vi "Dashboard Main.vi"() -> ()   [LabVIEW 2019]
uses:
  3750-Code-2020-Motion/Motion_Profiler_Class-master/MotionProfile_MP_Class_Status.ctl
  3750-Code-2020-Motion/Motion_Profiler_Class-master/MotionProfile_TalonSetValueEnum.ctl
  <vilib>/Rock Robotics/Network Tables/NT Read Variant.vi
  <vilib>/Rock Robotics/Network Tables/NT Read Number.vi
  <vilib>/Rock Robotics/Network Tables/NT Write Number.vi
  <vilib>/Rock Robotics/Network Tables/NT Write Boolean.vi
  <vilib>/Rock Robotics/Network Tables/NT Write String.vi
  3750-Code-2020-Motion/Motion_Profiler_Class-master/MotionProfiles.lvclass
panel:
  in  "Tab Control":enum32{"MP", "Shooter", "Drivetrain"}(tab)
  in  "Auto Selector":string(combo)
  in  "Start Logging":bool
  out "Right Motor":T1(graph)
  out "Right Throttle":dbl(graph)
  out "Left Throttle":dbl(graph)
  out "Left Motor":T2(graph)
  out "Left Bottom Buf Count":i32
  out "Left Under Run":bool
  out "Right Under Run":bool
  out "Right Bottom Buf Count":i32
  out "Turret Position":cluster{dbl, dbl}(knob) scale=-2000.0..2000.0
  out "Waveform Chart":cluster{"Numeric":dbl, "Numeric":dbl}(graph)
  in  "Set PID":bool
  in  "D":dbl
  in  "I":dbl
  in  "P":dbl
  in  "TCP":refnum<k5>
  out "Robot IP":string
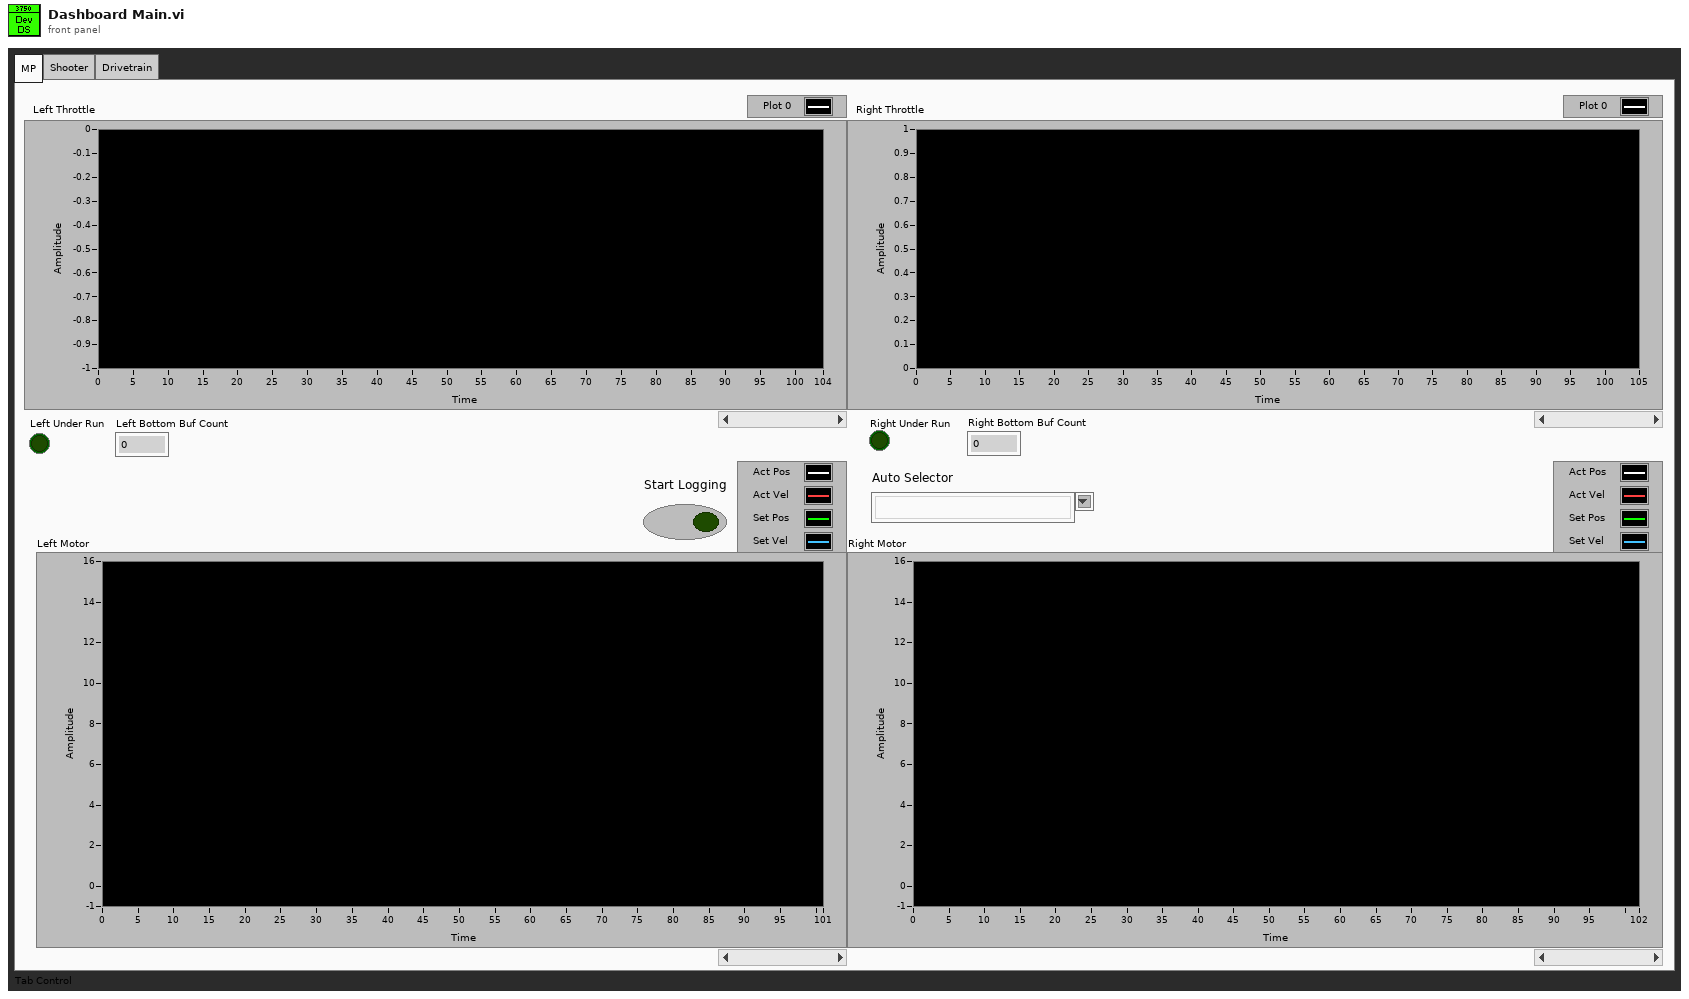
[diagram p1: front panel]
types:
  T1 = cluster{"Set_Vel_(u/100ms)":i32, "Act_Vel_(u/100ms)":i32, "Set_Pos_(u)":i32, "Act_Pos(u)":i32}
  T2 = cluster{"Set_Pos_(u)":i32, "Set_Pos_(u)":i32, "Act_Vel_(u/100ms)":i32, "Set_Vel_(u/100ms)":i32}
  T3 = cluster{"Error Strings":string, "Disable Counts":cluster{u16, u16}, "Rail Faults":cluster{u16, u16, u16}, "Robot IP":string, "DB Mode":u8, "Event Info":cluster{"Name":string, "Type":u8, "Number":u16, "Replay":u8}}
  T4 = cluster{"Storage":cluster{"Disk Free":u64, "RAM Block":u32, "RAM free":u32}, "CPU Utilization":cluster{"CPU % ISR":sgl, "CPU % Time Crit":sgl, "CPU % Timed Str":sgl, "CPU % High":sgl, "CPU % Above":sgl, "CPU % Normal":sgl, "CPU % Low":sgl}, "CAN":cluster{"% Bus Utilization":sgl, "Bus Off Cnt":u32, "TX_FIFO Full Cnt":u32, "Receive Error Cnt":u8, "Transmit Error Cnt":u8}, "HID":cluster{"HID Outputs":u32, "Rumble Low":u16, "Rumble High":u16}[]}
  T5 = cluster{"Status bits":cluster{"Test Mode":bool, "Autonomous":bool, "Enabled":bool, "Code Start":bool, "Brownout":bool, "Reserved 2":bool, "Reserved 3":bool, "E-Stop":bool}, "Code Trace":cluster{"Disabled":bool, "TeleOp":bool, "Auto":bool, "Test":bool}, "Controller Type":enum16{"unknown", "cRIO", "roboRio"}, "Code?":enum16{"unknown", "noCode", "code"}, "Battery V":dbl}
  T6 = cluster{"Control Bits":cluster{"TestMode":bool, "Autonomous":bool, "Enabled":bool, "FMS Present":bool, bool, bool, bool, "E-Stop":bool}, "Team Station ":u8, "Countdown":sgl, "Joystick Values":cluster{"Axes":dbl[], "Buttons":bool[], "POVs":i16[]}[]}
  T7 = enum8{"Tele-Op Disabled", "Tele-Op Enabled", "Auto Disabled", "Auto Enabled", "Test Disabled", "Test Enabled", "Disconnected", "No Code", "E-Stop"}
  T8 = typedef "MotionProfiles.lvclass/MotionProfile_MP_Class_Status.ctl" = cluster{"Motion Profile Status":cluster{"Top Buffer Remaining":i32, "Top Buffer Count":i32, "Bottom Buffer Count":i32, "Has Underrun?":bool, "Is Underrun?":bool, "Active Point Valid?":bool, "Is Last?":bool, "Profile Slot Select 0":i32, "Output Enable":i32, "Time Duration (ms)":i32, "Profile Slot Select 1":i32}, "TalonState":T9, "MP Is Done":bool, "MP Is Executing":bool, "Set_Vel_(u/100ms)":i32, "Set_Pos_(u)":i32, "Act_Vel_(u/100ms)":i32, "Act_Pos(u)":i32, "Throtle":dbl}
  T9 = typedef "MotionProfiles.lvclass/MotionProfile_TalonSetValueEnum.ctl" = enum16{"Disable", "Enable", "Hold"}
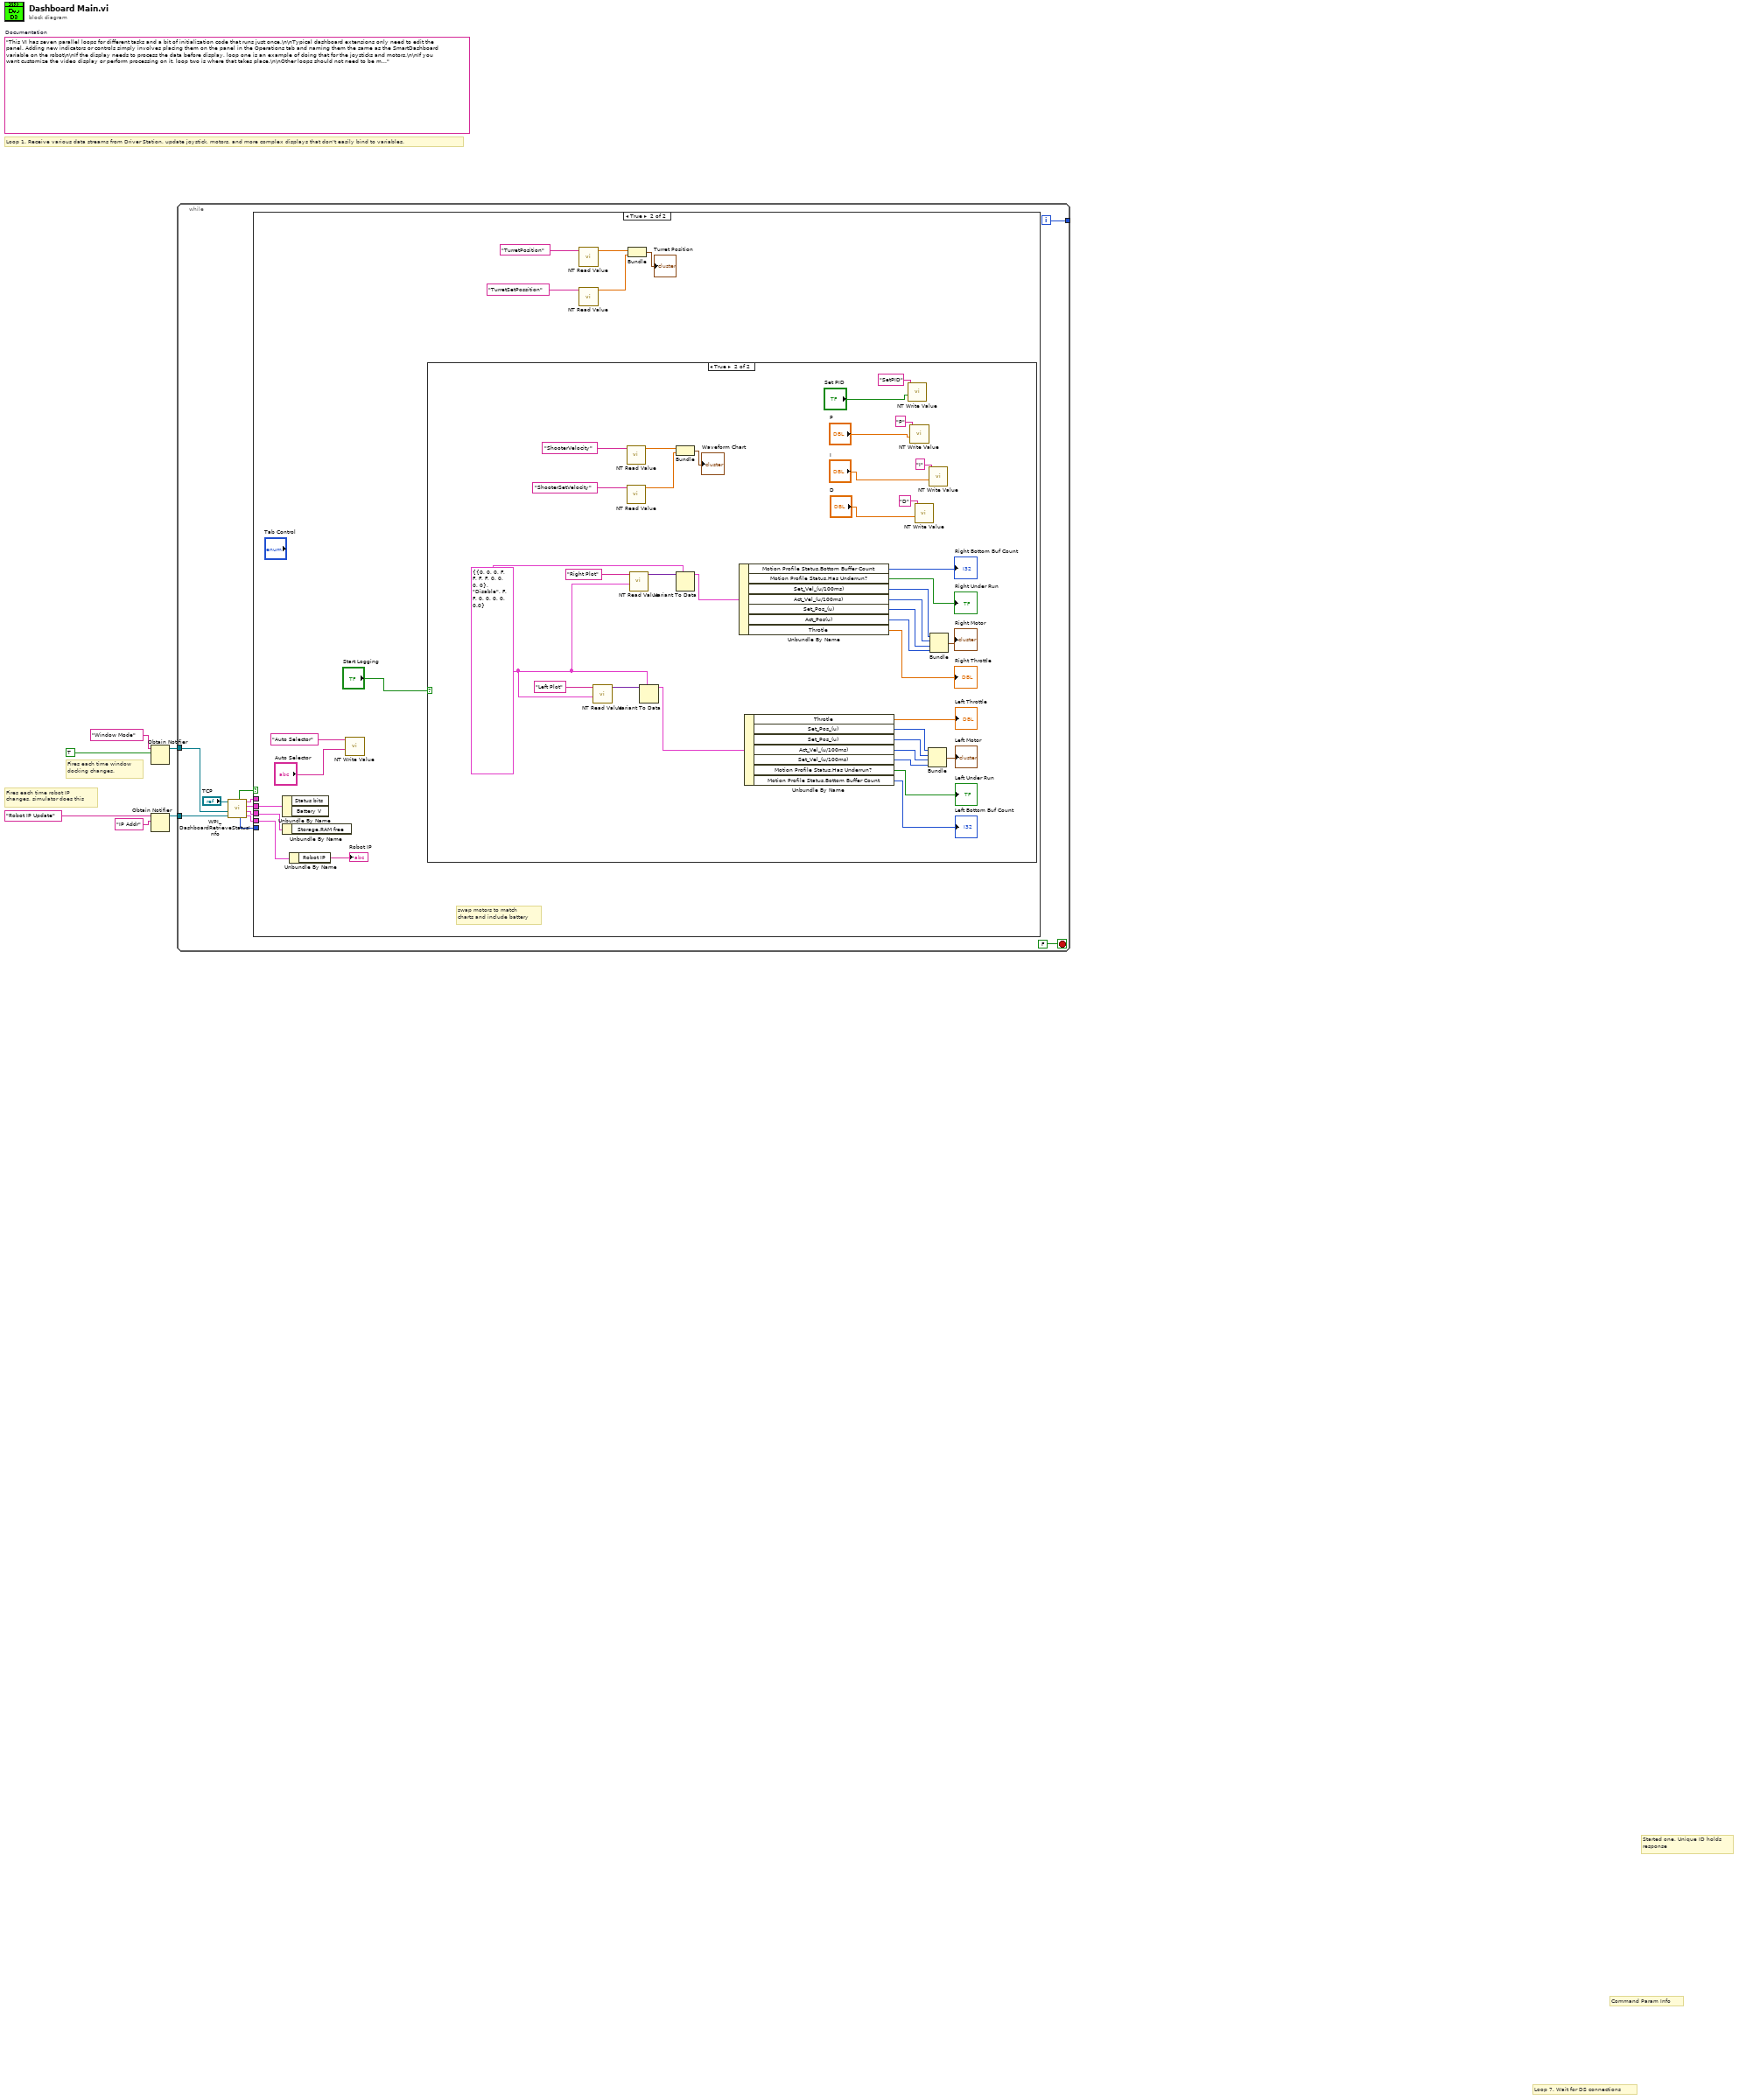
[diagram p0: block diagram]
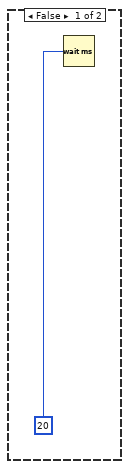
[diagram p2: hidden frame]
diagram:
  (unwired) "This VI has seven parallel loops for different tasks and a bit of initialization code that runs just once.\n\nTypical dashboard extensions only need to edit the panel. Adding new indicators or controls simply involves placing them on the panel in the Operations tab and naming them the same as the SmartDashboard variable on the robot\n\nIf the display needs to process the data before display, loop one is an example of doing that for the joysticks and motors.\n\nIf you want customize the video display or perform processing on it, loop two is where that takes place.\n\nOther loops should not need to be modified. They are pretty standard, and document the task they perform."  # Documentation
  # "Command Param Info"
  # "Started one, Unique ID holds\nresponse"
  # "Loop 7. Wait for DS connections"
  # "Fires each time robot IP\nchanges, simulator does this"
  # "Fires each time window\ndocking changes."
  # "Loop 1. Receive various data streams from Driver Station, update joystick, motors, and more complex displays that don't easily bind to variables."
  n1 = Obtain Notifier(name (unnamed)="Window Mode", notification data type=TRUE) -> (notifier out=w1:refnum<notifier>)  [unwired: 2 in, 2 out]
  n2 = Obtain Notifier(name (unnamed)="Robot IP Update", notification data type="IP Addr" ("name (unnamed)")) -> (notifier out=w2:refnum<notifier>)  [unwired: 2 in, 2 out]
  n3 = while {
    tunnel: [w17] -> _
    tunnel: w2 -> [w11]
    tunnel: w1 -> [w8]
    i -> [w17]
    stop <- FALSE stop-if-true
    n4 = call <vilib>:"WPI_DashboardRetrieveStatusInfo.vi"("Binding Refnum"=w11, "Window Mode Notifier"=w8, "TCP Cnx"="TCP") -> ("Power and Errors"=w12:T3, "Robot Metrics"=w15:T4, "Status Info"=w16:T5, "Control Info"=w13:T6, "Robot Mode"=w10:T7, "Process?"=w14:bool)  [unwired: 3 in]
    n5 = case shown="True" w14 {
      tunnel: w16 -> [_ w30]
      tunnel: w15 -> [_ w29]
      tunnel: w13 -> [_ _]
      tunnel: w12 -> [_ w28]
      tunnel: w10 -> [_ _]
      frame False {
        n6 = Wait (ms)(milliseconds to wait=u32 20) -> ()  [unwired: 1 out]
      }
      frame True {
        # "swap motors to match\ncharts and include battery"
        n7 = Unbundle By Name(w30) -> ()  [unwired: 2 out]
        n8 = Unbundle By Name(w29) -> ()  [unwired: 1 out]
        n9 = Unbundle By Name(w28) -> ("Robot IP"=→"Robot IP":string)
        n10 = call-poly <vilib>:"NT Write Value.vi"("String"="Auto Selector", "Name"="Auto Selector") -> ()  [unwired: 9 in, 1 out]
        n11 = case shown="True" "Start Logging" {
          frame False {
          }
          frame True {
            w62 = T8 {"Motion Profile Status"={"Top Buffer Remaining"=0, "Top Buffer Count"=0, "Bottom Buffer Count"=0, "Has Underrun?"=FALSE, "Is Underrun?"=FALSE, "Active Point Valid?"=FALSE, "Is Last?"=FALSE, "Profile Slot Select 0"=0, "Output Enable"=0, "Time Duration (ms)"=0, "Profile Slot Select 1"=0}, "TalonState"=enum."Disable", "MP Is Done"=FALSE, "MP Is Executing"=FALSE, "Set_Vel_(u/100ms)"=0, "Set_Pos_(u)"=0, "Act_Vel_(u/100ms)"=0, "Act_Pos(u)"=0, "Throtle"=0.0} ("MP_Class_Status")
            n12 = call-poly <vilib>:"NT Read Value.vi"("Default Value"=w62, "Name"="Left Plot") -> ("Variant"=w63:variant)  [unwired: 8 in, 1 out]
            n13 = call-poly <vilib>:"NT Read Value.vi"("Name"="ShooterVelocity") -> ("Numeric"=w42:dbl)  [unwired: 9 in, 1 out]
            n14 = call-poly <vilib>:"NT Read Value.vi"("Name"="ShooterSetVelocity") -> ("Numeric"=w43:dbl)  [unwired: 9 in, 1 out]
            n15 = call-poly <vilib>:"NT Read Value.vi"("Default Value"=w62, "Name"="Right Plot") -> ("Variant"=w65:variant)  [unwired: 8 in, 1 out]
            n16 = Variant To Data(type=w62, Variant=w63) -> (data=w44:T8)  [unwired: 1 in, 1 out]
            n17 = Bundle("Numeric"=w42, "Numeric"=w43) -> (→"Waveform Chart":cluster{"Numeric":dbl, "Numeric":dbl})  [unwired: 1 in]
            n18 = Variant To Data(type=w62, Variant=w65) -> (data=w53:T8)  [unwired: 1 in, 1 out]
            n19 = Unbundle By Name(w53) -> ("Motion Profile Status.Bottom Buffer Count"=→"Right Bottom Buf Count":i32, "Motion Profile Status.Has Underrun?"=→"Right Under Run":bool, "Set_Vel_(u/100ms)"=w58:i32, "Act_Vel_(u/100ms)"=w57:i32, "Set_Pos_(u)"=w56:i32, "Act_Pos(u)"=w55:i32, "Throtle"=→"Right Throttle":dbl)
            n20 = Unbundle By Name(w44) -> ("Throtle"=→"Left Throttle":dbl, "Set_Pos_(u)"=w46:i32, "Set_Pos_(u)"=w47:i32, "Act_Vel_(u/100ms)"=w48:i32, "Set_Vel_(u/100ms)"=w49:i32, "Motion Profile Status.Has Underrun?"=→"Left Under Run":bool, "Motion Profile Status.Bottom Buffer Count"=→"Left Bottom Buf Count":i32)
            n21 = call-poly <vilib>:"NT Write Value.vi"("Boolean"="Set PID", "Name"="SetPID") -> ()  [unwired: 9 in, 1 out]
            n22 = call-poly <vilib>:"NT Write Value.vi"("Numeric"="P", "Name"="P") -> ()  [unwired: 9 in, 1 out]
            n23 = call-poly <vilib>:"NT Write Value.vi"("Numeric"="D", "Name"="D") -> ()  [unwired: 9 in, 1 out]
            n24 = Bundle("Set_Pos_(u)"=w46, "Set_Pos_(u)"=w47, "Act_Vel_(u/100ms)"=w48, "Set_Vel_(u/100ms)"=w49) -> (→"Left Motor":T2)  [unwired: 1 in]
            n25 = call-poly <vilib>:"NT Write Value.vi"("Numeric"="I", "Name"="I") -> ()  [unwired: 9 in, 1 out]
            n26 = Bundle("Set_Vel_(u/100ms)"=w58, "Act_Vel_(u/100ms)"=w57, "Set_Pos_(u)"=w56, "Act_Pos(u)"=w55) -> (→"Right Motor":T1)  [unwired: 1 in]
          }
        }
        n27 = call-poly <vilib>:"NT Read Value.vi"("Name"="TurretPosition") -> ("Numeric"=w22:dbl)  [unwired: 9 in, 1 out]
        n28 = call-poly <vilib>:"NT Read Value.vi"("Name"="TurretSetPossition") -> ("Numeric"=w21:dbl)  [unwired: 9 in, 1 out]
        n29 = Bundle("Numeric"=w22, "Numeric"=w21) -> (→"Turret Position":cluster{"Numeric":dbl, "Numeric":dbl})  [unwired: 1 in]
      }
    }
  }
